vi "NXTMMX-DM.vi"(0 "Input of Motor Multiplexer":T4={"NXTMMX Address"=6, "Which Motor"=0, "Operation"=0, "Next Action"=0, "Position"=0, "Direction"=FALSE, "Power"=100, "Durartion"=0, "Wait for Completion"=FALSE, "Relative"=FALSE} {"Next Action" items=["Float", "Brake"]; "Operation" items=["Run Unlimited", "Run Seconds", "Run Tachometer"]; "Which Motor" items=["Motor 1", "Motor 2", "Both Motors"]; "NXTMMX Address" min=2 max=254 step=2 format="%x"}, 2 "NXT":T2={"Hardware"="NXT", "Flattened String"=""}, 3 "Input Port":T3 items=["Port 1", "Port 2", "Port 3", "Port 4"]) -> (1 "Output of Motor Multiplexer":T1, 4 "NXT dup":T2={"Hardware"="NXT", "Flattened String"=""})   [LabVIEW 2010]
uses:
  <vilib>/NXT/Block Support/NXT_InputPort.ctl
  <vilib>/NXT/Subs/LVHSConnector.ctl
  <vilib>/NXT/Block Support/HWPage.SensorType.ctl
  <vilib>/NXT/Block Support/HWPage.SensorMode.ctl
  <vilib>/NXT/Dual Mode Library/Waits/Wait_Num(msec).vi
panel:
  out "Address":i32
  # "mindsensors.com\nCopyright (c) 2009 by mindsensors.com\nEmail: info (<at>) mindsensors (<dot>) com\n\nThis program is free software. You can redistribute it and/or modify\nit under the terms of the GNU General Public License as published by\nthe Free Software Foundation; version 3 of the License.\nRead the license at: http://www.gnu.org/licenses/gpl.txt"
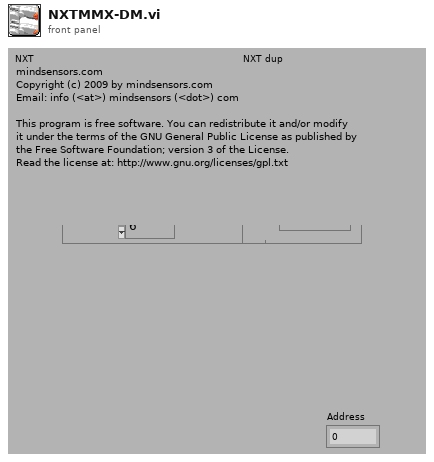
[diagram p1: front panel]
types:
  T1 = cluster{"Milivolts":u16, "Position 1":i32, "Position 2":i32, "Motor battery Voltage":dbl}
  T2 = typedef "LVHSConnector.ctl" = cluster{"Hardware":string, "Flattened String":string}
  T3 = typedef "NXT_InputPort.ctl" = u8
  T4 = cluster{"NXTMMX Address":u8, "Which Motor":u8, "Operation":u8, "Next Action":u8, "Position":i32, "Direction":bool, "Power":i8, "Durartion":u8, "Wait for Completion":bool, "Relative":bool}
  T5 = typedef "HWPage.SensorType.ctl" = u8
  T6 = typedef "HWPage.SensorMode.ctl" = u8
  T7 = cluster{"millivolts":i32, "(hi.lo)":u16, "(hi.lo)":u16, dbl}
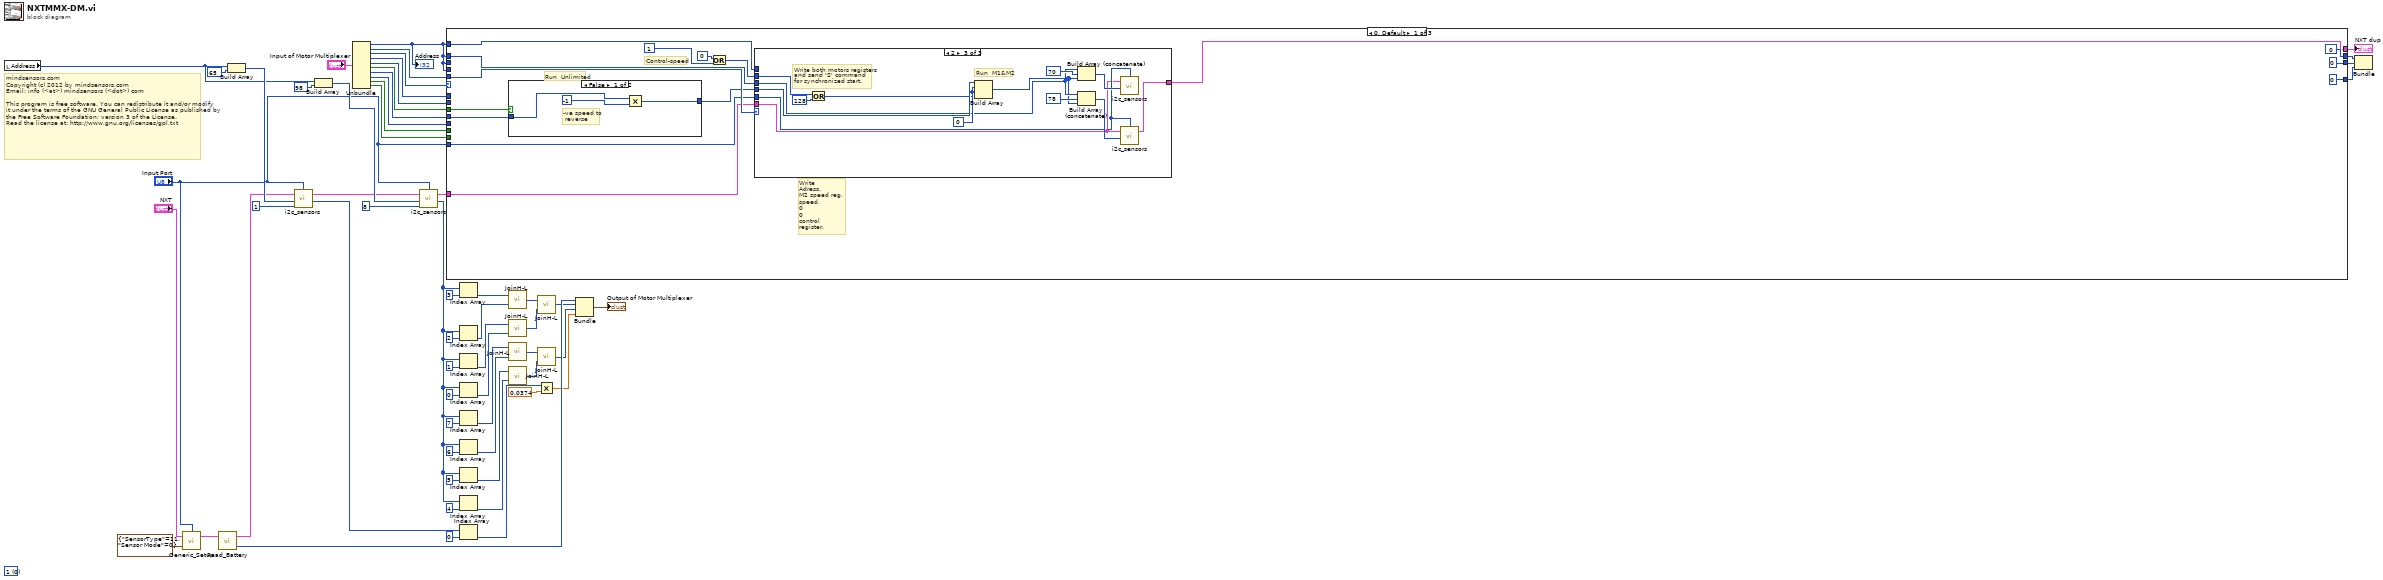
[diagram p0: block diagram]
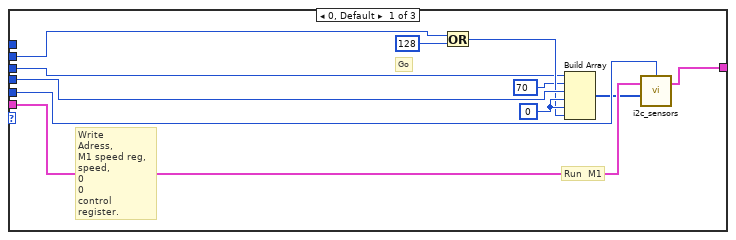
[diagram p2: hidden frame]
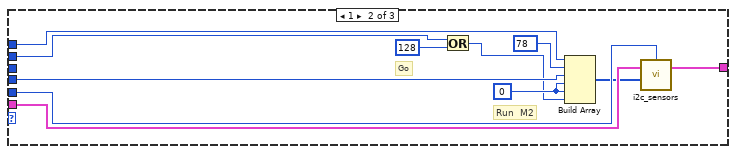
[diagram p3: hidden frame]
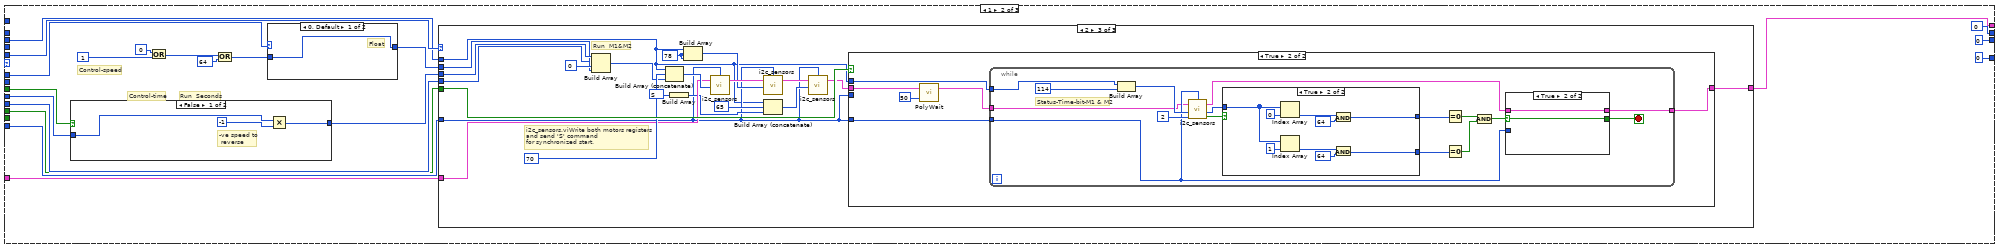
[diagram p5: hidden frame]
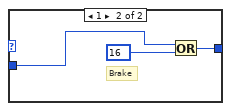
[diagram p6: hidden frame]
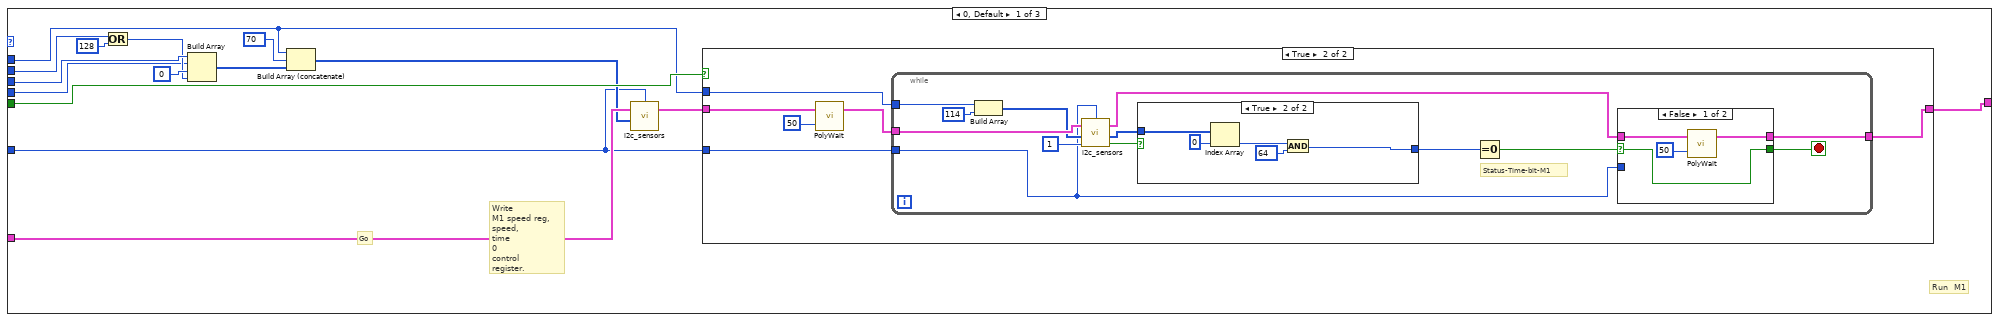
[diagram p7: hidden frame]
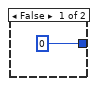
[diagram p10: hidden frame]
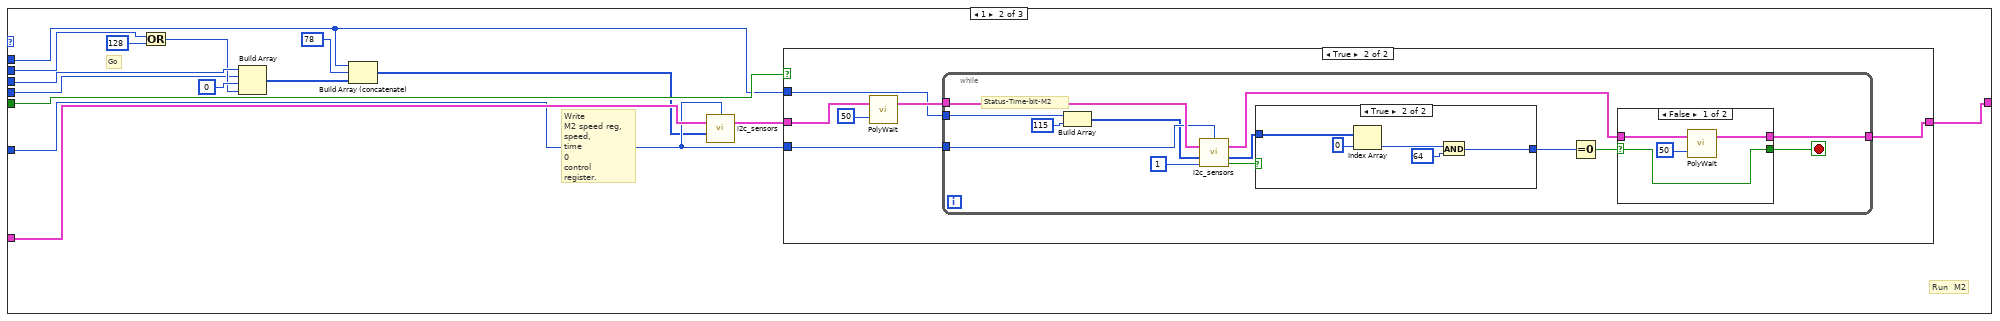
[diagram p11: hidden frame]
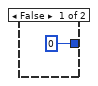
[diagram p14: hidden frame]
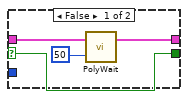
[diagram p16: hidden frame]
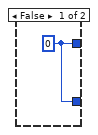
[diagram p17: hidden frame]
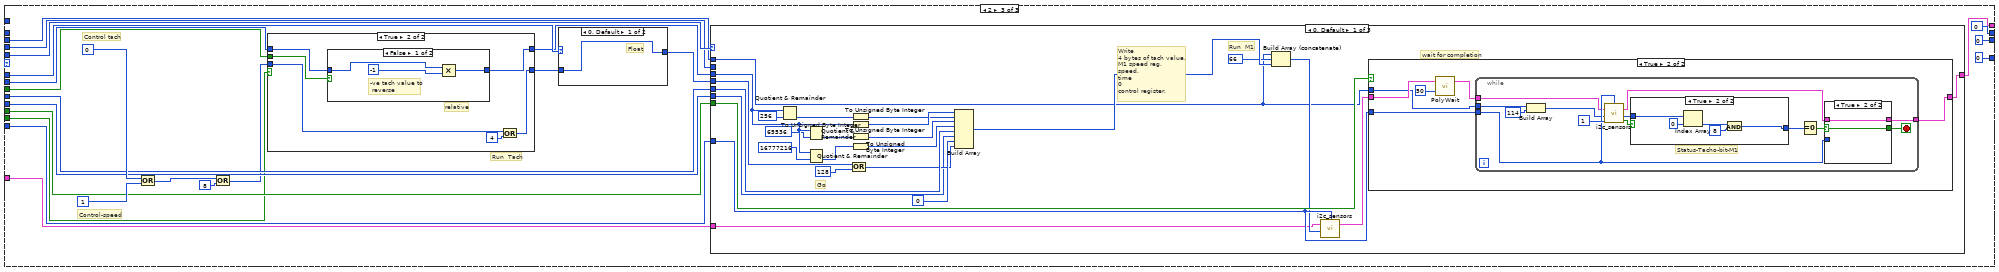
[diagram p19: hidden frame]
diagram:
  (unwired) i16 0 items=["1", "2", "3", "4", "5", "6", "7", "8"] ("Line")
  # "mindsensors.com\nCopyright (c) 2012 by mindsensors.com\nEmail: info (<at>) mindsensors (<dot>) com\n\nThis program is free software. You can redistribute it and/or modify\nit under the terms of the GNU General Public License as published by\nthe Free Software Foundation; version 3 of the License.\nRead the license at: http://www.gnu.org/licenses/gpl.txt"
  n1 = local read "Address"() -> (w4:i32)
  n2 = call <vilib>:"Generic_Setup.vi"("Sensor Setup"=cluster{"SensorType":T5, "Sensor Mode":T6} {"SensorType"=11, "Sensor Mode"=0}, "NXT"="NXT", "Port"="Input Port") -> ("NXT"=w49:T2)  [unwired: 1 out]
  n3 = call <vilib>:"Read_Battery.vi"("NXT"=w49) -> ("millivolts"=w23:i32, "NXT"=w3:T2)  [unwired: 2 in]
  n4 = Build Array(w4, u8 65 ("Reg Address")) -> (w35:i32[])
  n5 = call <vilib>:"i2c_sensors.vi"("Return Length"=u8 1 ("bytes to read"), "Bytes to Write"=w35, "NXT"=w3, "Port"="Input Port") -> ("Bytes read"=w34:u8[], "NXT"=w29:T2)  [unwired: 1 in, 1 out]
  n6 = Build Array(w4, u8 98 ("Reg Address")) -> (w33:i32[])
  n7 = Unbundle("Input of Motor Multiplexer") -> ("NXTMMX Address"=w51:u8, "Which Motor"=w53:u8, "Operation"=w58:u8, "Next Action"=w57:u8, "Position"=w55:i32, "Direction"=w54:bool, "Power"=w56:i8, "Durartion"=w52:u8, "Wait for Completion"=w25:bool, "Relative"=w24:bool)
  "Address" <- w51
  n8 = call <vilib>:"i2c_sensors.vi"("Return Length"=u8 8 ("bytes to read"), "Bytes to Write"=w33, "NXT"=w29, "Port"="Input Port") -> ("Bytes read"=w30:u8[], "NXT"=w27:T2)  [unwired: 1 in, 1 out]
  n9 = case shown="0, Default" w58 {
    tunnel: w54 -> [w72 w132 w318]
    tunnel: w56 -> [w71 w131 w308]
    tunnel: w53 -> [w70 w130 w317]
    tunnel: "Input Port" -> [w68 w128 w316]
    tunnel: w52 -> [_ w125 w313]
    tunnel: w57 -> [_ w124 w312]
    tunnel: w55 -> [_ _ w309]
    tunnel: w25 -> [_ w121 w310]
    tunnel: w24 -> [_ _ w306]
    tunnel: [0 0 0] -> w22
    tunnel: [u32 0 ("Out") u32 0 ("Out") u32 0 ("Out")] -> w21
    tunnel: [u16 0 u16 0 u16 0] -> w20
    tunnel: w27 -> [w63 w117 w299]
    tunnel: [w62 w116 w300] -> w19
    tunnel: w51 -> [_ w115 w298]
    tunnel: w51 -> [w61 _ _]
    tunnel: w51 -> [_ _ w297]
    tunnel: w51 -> [w60 _ _]
    frame 0, Default {
      # "Write\nAdress, \nM2 speed reg,\nspeed,\n0\n0\ncontrol register."
      # "Control-speed"
      # "Run  Unlimited"
      n10 = case shown="False" w72 {
        tunnel: w71 -> [w113 w114]
        tunnel: [w111 w114] -> w69
        frame False {
          # "-ve speed to\n reverse"
          n11 = Multiply(x=w113, y=i8 -1) -> (x*y=w111:i8)
        }
        frame True {
        }
      }
      n12 = Or(x=0, y=1) -> (x .or. y?=w67:i32)
      n13 = case shown="2" w70 {
        tunnel: w67 -> [w84 w95 w98]
        tunnel: w69 -> [w83 w94 w105]
        tunnel: w68 -> [w78 w91 w102]
        tunnel: w63 -> [w80 w90 w101]
        tunnel: [w79 w89 w100] -> w62
        tunnel: w61 -> [w77 _ w104]
        tunnel: w60 -> [_ w88 _]
        frame 0, Default {
          w82 = 0
          # "Go"
          # "Run  M1"
          # "Write \nAdress,\nM1 speed reg,\nspeed,\n0\n0\ncontrol register."
          n14 = Or(x=w84, y=128) -> (x .or. y?=w81:i32)
          n15 = Build Array(w77, 70, w83, w82, w82, w81) -> (w75:i32[])
          n16 = call <vilib>:"i2c_sensors.vi"("Bytes to Write"=w75, "NXT"=w80, "Port"=w78) -> ("NXT"=w79:T2)  [unwired: 2 in, 2 out]
        }
        frame 1 {
          w93 = 0
          # "Go"
          # "Run  M2"
          n17 = Or(x=w95, y=128) -> (x .or. y?=w92:i32)
          n18 = Build Array(w88, 78, w94, w93, w93, w92) -> (w86:i32[])
          n19 = call <vilib>:"i2c_sensors.vi"("Bytes to Write"=w86, "NXT"=w90, "Port"=w91) -> ("NXT"=w89:T2)  [unwired: 2 in, 2 out]
        }
        frame 2 {
          w106 = 0
          # "Write both motors registers\nand send 'S' command \nfor synchronized start."
          # "Run  M1&M2"
          n20 = Or(x=w98, y=128) -> (x .or. y?=w97:i32)
          n21 = Build Array(w105, w106, w106, w97) -> (w103:i32[])
          n22 = Build Array (concatenate)(w104, 70, w103) -> (w107:i32[])
          n23 = Build Array (concatenate)(w104, 78, w103) -> (w109:i32[])
          n24 = call <vilib>:"i2c_sensors.vi"("Bytes to Write"=w107, "NXT"=w101, "Port"=w102) -> ()  [unwired: 2 in, 3 out]
          n25 = call <vilib>:"i2c_sensors.vi"("Bytes to Write"=w109, "NXT"=w101, "Port"=w102) -> ("NXT"=w100:T2)  [unwired: 2 in, 2 out]
        }
      }
    }
    frame 1 {
      # "Control-time"
      # "Control-speed"
      # "Run  Seconds"
      n26 = case shown="False" w132 {
        tunnel: w131 -> [w295 w296]
        tunnel: [w293 w296] -> w129
        frame False {
          # "-ve speed to\n reverse"
          n27 = Multiply(x=w295, y=i8 -1) -> (x*y=w293:i8)
        }
        frame True {
        }
      }
      n28 = Or(x=0, y=1) -> (x .or. y?=w126:i32)
      n29 = Or(x=w126, y=64) -> (x .or. y?=w123:i32)
      n30 = case shown="0, Default" w124 {
        tunnel: w123 -> [w135 w137]
        tunnel: [w135 w138] -> w122
        frame 0, Default {
          # "Float"
        }
        frame 1 {
          # "Brake"
          n31 = Or(x=w137, y=16) -> (x .or. y?=w138:i32)
        }
      }
      n32 = case shown="2" w130 {
        tunnel: w122 -> [w152 w199 w250]
        tunnel: w129 -> [w151 w198 w253]
        tunnel: w128 -> [w141 w190 w235]
        tunnel: w125 -> [w148 w195 w249]
        tunnel: w121 -> [w147 w194 w248]
        tunnel: w117 -> [w145 w193 w244]
        tunnel: [w140 w187 w234] -> w116
        tunnel: w115 -> [w139 w186 w233]
        frame 0, Default {
          # "Go"
          # "Run  M1"
          # "Write \nM1 speed reg,\nspeed,\ntime\n0\ncontrol register."
          n33 = Or(x=w152, y=128) -> (x .or. y?=w149:i32)
          n34 = Build Array(w151, w148, 0, w149) -> (w142:i32[])
          n35 = Build Array (concatenate)(w139, 70, w142) -> (w144:i32[])
          n36 = call <vilib>:"i2c_sensors.vi"("Bytes to Write"=w144, "NXT"=w145, "Port"=w141) -> ("NXT"=w146:T2)  [unwired: 2 in, 2 out]
          n37 = case shown="True" w147 {
            tunnel: w141 -> [_ w160]
            tunnel: w146 -> [w154 w158]
            tunnel: [w154 w156] -> w140
            tunnel: w139 -> [_ w155]
            frame False {
            }
            frame True {
              n38 = call-poly <vilib>:"PolyWait.vi"("Time (100 msec)"=u16 50 ("Delay ms"), "NXT"=w158) -> ("NXT"=w157:T2)  [unwired: 2 in]
              n39 = while {
                tunnel: w160 -> [w164]
                tunnel: w157 -> [w169]
                tunnel: [w168] -> w156
                tunnel: w155 -> [w162]
                stop <- w172 stop-if-true
                # "Status-Time-bit-M1"
                n40 = Build Array(w162, 114) -> (w165:i32[])
                n41 = call <vilib>:"i2c_sensors.vi"("Return Length"=1, "Bytes to Write"=w165, "NXT"=w169, "Port"=w164) -> ("Success?"=w161:bool, "Bytes read"=w167:u8[], "NXT"=w170:T2)  [unwired: 1 in]
                n42 = case shown="True" w161 {
                  tunnel: w167 -> [_ w185]
                  tunnel: [u8 0 w181] -> w173
                  frame False {
                  }
                  frame True {
                    n43 = Index Array(array=w185, index=0) -> (element=w182:u8)
                    n44 = And(x=w182, y=u8 64) -> (x .and. y?=w181:u8)
                  }
                }
                n45 = Equal To 0?(x=w173) -> (x = 0?=w171:bool)
                n46 = case shown="False" w171 {
                  selector: w171 -> [w177 w179]
                  tunnel: w164 -> [_ _]
                  tunnel: [w177 w179] -> w172
                  tunnel: w170 -> [w175 w178]
                  tunnel: [w174 w178] -> w168
                  frame False {
                    n47 = call-poly <vilib>:"PolyWait.vi"("Time (100 msec)"=u16 50 ("Delay ms"), "NXT"=w175) -> ("NXT"=w174:T2)  [unwired: 2 in]
                  }
                  frame True {
                  }
                }
              }
            }
          }
        }
        frame 1 {
          # "Go"
          # "Run  M2"
          # "Write \nM2 speed reg,\nspeed,\ntime\n0\ncontrol register."
          n48 = Or(x=w199, y=128) -> (x .or. y?=w196:i32)
          n49 = Build Array(w198, w195, 0, w196) -> (w191:i32[])
          n50 = Build Array (concatenate)(w186, 78, w191) -> (w189:i32[])
          n51 = call <vilib>:"i2c_sensors.vi"("Bytes to Write"=w189, "NXT"=w193, "Port"=w190) -> ("NXT"=w188:T2)  [unwired: 2 in, 2 out]
          n52 = case shown="True" w194 {
            tunnel: w190 -> [_ w207]
            tunnel: w188 -> [w201 w205]
            tunnel: [w201 w203] -> w187
            tunnel: w186 -> [_ w202]
            frame False {
            }
            frame True {
              n53 = call-poly <vilib>:"PolyWait.vi"("Time (100 msec)"=u16 50 ("Delay ms"), "NXT"=w205) -> ("NXT"=w204:T2)  [unwired: 2 in]
              n54 = while {
                tunnel: w207 -> [w214]
                tunnel: w204 -> [w215]
                tunnel: [w217] -> w203
                tunnel: w202 -> [w209]
                stop <- w219 stop-if-true
                # "Status-Time-bit-M2"
                n55 = Build Array(w209, 115) -> (w211:i32[])
                n56 = call <vilib>:"i2c_sensors.vi"("Return Length"=1, "Bytes to Write"=w211, "NXT"=w215, "Port"=w214) -> ("Success?"=w208:bool, "Bytes read"=w210:u8[], "NXT"=w216:T2)  [unwired: 1 in]
                n57 = case shown="True" w208 {
                  tunnel: w210 -> [_ w232]
                  tunnel: [u8 0 w228] -> w220
                  frame False {
                  }
                  frame True {
                    n58 = Index Array(array=w232, index=0) -> (element=w229:u8)
                    n59 = And(x=w229, y=u8 64) -> (x .and. y?=w228:u8)
                  }
                }
                n60 = Equal To 0?(x=w220) -> (x = 0?=w218:bool)
                n61 = case shown="False" w218 {
                  selector: w218 -> [w224 w226]
                  tunnel: [w224 w226] -> w219
                  tunnel: [w222 w225] -> w217
                  tunnel: w216 -> [w221 w225]
                  frame False {
                    n62 = call-poly <vilib>:"PolyWait.vi"("Time (100 msec)"=u16 50 ("Delay ms"), "NXT"=w221) -> ("NXT"=w222:T2)  [unwired: 2 in]
                  }
                  frame True {
                  }
                }
              }
            }
          }
        }
        frame 2 {
          w251 = u16 83 items=["S"=83]
          w243 = 78
          # "i2c_sensors.viWrite both motors registers\nand send 'S' command \nfor synchronized start."
          # "Run  M1&M2"
          n63 = Build Array(w253, w249, 0, w250) -> (w246:i32[])
          n64 = Build Array (concatenate)(w233, 70, w246) -> (w245:i32[])
          n65 = Build Array(w251) -> (w241:u16[])
          n66 = Build Array(w233, w243, w243) -> (w238:i32[])
          n67 = call <vilib>:"i2c_sensors.vi"("Bytes to Write"=w245, "NXT"=w244, "Port"=w235) -> ("NXT"=w239:T2)  [unwired: 2 in, 2 out]
          n68 = call <vilib>:"i2c_sensors.vi"("Bytes to Write"=w238, "NXT"=w239, "Port"=w235) -> ("NXT"=w240:T2)  [unwired: 2 in, 2 out]
          n69 = Build Array (concatenate)(w233, 65, w241) -> (w237:i32[])
          n70 = call <vilib>:"i2c_sensors.vi"("Bytes to Write"=w237, "NXT"=w240, "Port"=w235) -> ("NXT"=w236:T2)  [unwired: 2 in, 2 out]
          n71 = case shown="True" w248 {
            tunnel: w235 -> [_ _]
            tunnel: w236 -> [w254 w259]
            tunnel: w235 -> [_ w257]
            tunnel: [w254 w256] -> w234
            tunnel: w233 -> [_ w255]
            frame False {
            }
            frame True {
              n72 = call-poly <vilib>:"PolyWait.vi"("Time (100 msec)"=u16 50 ("Delay ms"), "NXT"=w259) -> ("NXT"=w258:T2)  [unwired: 2 in]
              n73 = while {
                tunnel: w258 -> [w264]
                tunnel: w257 -> [w267]
                tunnel: [w263] -> w256
                tunnel: w255 -> [w262]
                stop <- w271 stop-if-true
                # "Status-Time-bit-M1 & M2"
                n74 = Build Array(w262, 114) -> (w268:i32[])
                n75 = call <vilib>:"i2c_sensors.vi"("Return Length"=2, "Bytes to Write"=w268, "NXT"=w264, "Port"=w267) -> ("Success?"=w261:bool, "Bytes read"=w266:u8[], "NXT"=w265:T2)  [unwired: 1 in]
                n76 = case shown="True" w261 {
                  tunnel: w266 -> [_ w291]
                  tunnel: [w283 w284] -> w276
                  tunnel: [w283 w286] -> w275
                  frame False {
                    w283 = u8 0
                  }
                  frame True {
                    n77 = Index Array(array=w291, index=0) -> (element=w287:u8)
                    n78 = Index Array(array=w291, index=1) -> (element=w285:u8)
                    n79 = And(x=w287, y=u8 64) -> (x .and. y?=w286:u8)
                    n80 = And(x=w285, y=u8 64) -> (x .and. y?=w284:u8)
                  }
                }
                n81 = Equal To 0?(x=w275) -> (x = 0?=w274:bool)
                n82 = Equal To 0?(x=w276) -> (x = 0?=w273:bool)
                n83 = And(x=w274, y=w273) -> (x .and. y?=w272:bool)
                n84 = case shown="True" w272 {
                  selector: w272 -> [w280 w282]
                  tunnel: w267 -> [_ _]
                  tunnel: [w280 w282] -> w271
                  tunnel: w265 -> [w278 w281]
                  tunnel: [w277 w281] -> w263
                  frame False {
                    n85 = call-poly <vilib>:"PolyWait.vi"("Time (100 msec)"=u16 50 ("Delay ms"), "NXT"=w278) -> ("NXT"=w277:T2)  [unwired: 2 in]
                  }
                  frame True {
                  }
                }
              }
            }
          }
        }
      }
    }
    frame 2 {
      # "Run  Tach"
      # "Control tach"
      # "Control-speed"
      n86 = Or(x=0, y=1) -> (x .or. y?=w314:i32)
      n87 = Or(x=w314, y=8) -> (x .or. y?=w305:i32)
      n88 = case shown="True" w306 {
        tunnel: w318 -> [_ w328]
        tunnel: w309 -> [w322 w327]
        tunnel: [w322 w326] -> w307
        tunnel: w305 -> [w321 w325]
        tunnel: [w321 w323] -> w304
        frame False {
          # "absolute\nignore the direction"
        }
        frame True {
          # "relative"
          n89 = case shown="False" w328 {
            tunnel: w327 -> [w331 w332]
            tunnel: [w329 w332] -> w326
            frame False {
              # "-ve tach value to\n reverse"
              n90 = Multiply(x=w331, y=i8 -1) -> (x*y=w329:i32)
            }
            frame True {
            }
          }
          n91 = Or(x=w325, y=4) -> (x .or. y?=w323:i32)
        }
      }
      n92 = case shown="0, Default" w312 {
        tunnel: [w333 w336] -> w311
        tunnel: w304 -> [w333 w334]
        frame 0, Default {
          # "Float"
        }
        frame 1 {
          # "Brake"
          n93 = Or(x=w334, y=16) -> (x .or. y?=w336:i32)
        }
      }
      n94 = case shown="0, Default" w317 {
        tunnel: w311 -> [w361 w419 w482]
        tunnel: w316 -> [w343 w400 w454]
        tunnel: w313 -> [w357 w415 w481]
        tunnel: w310 -> [w356 w414 w480]
        tunnel: w308 -> [w360 w418 w479]
        tunnel: w307 -> [w354 w407 w472]
        tunnel: [w337 w395 w467] -> w300
        tunnel: w299 -> [w340 w398 w466]
        tunnel: w298 -> [w338 _ _]
        tunnel: w297 -> [_ w396 _]
        frame 0, Default {
          # "wait for completion"
          # "Go"
          # "Run  M1"
          # "Write\n4 bytes of tach value. \nM1 speed reg,\nspeed,\ntime\n0\ncontrol register."
          n95 = Quotient & Remainder(x=w354, y=u32 256) -> (floor(x/y)=w350:u32)  [unwired: 1 out]
          n96 = Quotient & Remainder(x=w354, y=u32 65536) -> (floor(x/y)=w348:u32)  [unwired: 1 out]
          n97 = Quotient & Remainder(x=w354, y=u32 16777216) -> (floor(x/y)=w345:u32)  [unwired: 1 out]
          n98 = Or(x=w361, y=128) -> (x .or. y?=w358:i32)
          n99 = To Unsigned Byte Integer(number=w350) -> (unsigned 8bit integer=w349:u8)
          n100 = To Unsigned Byte Integer(number=w354) -> (unsigned 8bit integer=w355:u8)
          n101 = To Unsigned Byte Integer(number=w348) -> (unsigned 8bit integer=w347:u8)
          n102 = To Unsigned Byte Integer(number=w345) -> (unsigned 8bit integer=w346:u8)
          n103 = Build Array(w355, w349, w347, w346, w360, w357, 0, w358) -> (w344:i32[])
          n104 = Build Array (concatenate)(w338, 66, w344) -> (w341:i32[])
          n105 = call <vilib>:"i2c_sensors.vi"("Bytes to Write"=w341, "NXT"=w340, "Port"=w343) -> ("NXT"=w339:T2)  [unwired: 2 in, 2 out]
          n106 = case shown="True" w356 {
            tunnel: w343 -> [_ w369]
            tunnel: w339 -> [w363 w367]
            tunnel: w338 -> [_ w366]
            tunnel: [w363 w364] -> w337
            frame False {
            }
            frame True {
              n107 = call-poly <vilib>:"PolyWait.vi"("Time (100 msec)"=u16 50 ("Delay ms"), "NXT"=w367) -> ("NXT"=w365:T2)  [unwired: 2 in]
              n108 = while {
                tunnel: w369 -> [w377]
                tunnel: w366 -> [w375]
                tunnel: w365 -> [w374]
                tunnel: [w372] -> w364
                stop <- w380 stop-if-true
                # "Status-Tacho-bit-M1"
                n109 = Build Array(w375, 114) -> (w370:i32[])
                n110 = call <vilib>:"i2c_sensors.vi"("Return Length"=1, "Bytes to Write"=w370, "NXT"=w374, "Port"=w377) -> ("Success?"=w371:bool, "Bytes read"=w378:u8[], "NXT"=w373:T2)  [unwired: 1 in]
                n111 = case shown="True" w371 {
                  tunnel: w378 -> [_ w394]
                  tunnel: [u8 0 w390] -> w382
                  frame False {
                  }
                  frame True {
                    n112 = Index Array(array=w394, index=0) -> (element=w391:u8)
                    n113 = And(x=w391, y=u8 8) -> (x .and. y?=w390:u8)
                  }
                }
                n114 = Equal To 0?(x=w382) -> (x = 0?=w381:bool)
                n115 = case shown="True" w381 {
                  selector: w381 -> [w386 w388]
                  tunnel: w377 -> [_ _]
                  tunnel: [w386 w388] -> w380
                  tunnel: w373 -> [w384 w387]
                  tunnel: [w383 w387] -> w372
                  frame False {
                    n116 = call-poly <vilib>:"PolyWait.vi"("Time (100 msec)"=u16 50 ("Delay ms"), "NXT"=w384) -> ("NXT"=w383:T2)  [unwired: 2 in]
                  }
                  frame True {
                  }
                }
              }
            }
          }
        }
        frame 1 {
          # "Go"
          # "Run  M2"
          # "Write \nM2 speed reg,\nspeed,\ntime\n0\ncontrol register."
          n117 = Quotient & Remainder(x=w407, y=u32 256) -> (floor(x/y)=w410:u32)  [unwired: 1 out]
          n118 = Quotient & Remainder(x=w407, y=u32 65536) -> (floor(x/y)=w409:u32)  [unwired: 1 out]
          n119 = Quotient & Remainder(x=w407, y=u32 16777216) -> (floor(x/y)=w408:u32)  [unwired: 1 out]
          n120 = Or(x=w419, y=128) -> (x .or. y?=w416:i32)
          n121 = To Unsigned Byte Integer(number=w410) -> (unsigned 8bit integer=w405:u8)
          n122 = To Unsigned Byte Integer(number=w407) -> (unsigned 8bit integer=w406:u8)
          n123 = To Unsigned Byte Integer(number=w409) -> (unsigned 8bit integer=w404:u8)
          n124 = To Unsigned Byte Integer(number=w408) -> (unsigned 8bit integer=w403:u8)
          n125 = Build Array(w406, w405, w404, w403, w418, w415, 0, w416) -> (w401:i32[])
          n126 = Build Array (concatenate)(w396, 74, w401) -> (w399:i32[])
          n127 = call <vilib>:"i2c_sensors.vi"("Bytes to Write"=w399, "NXT"=w398, "Port"=w400) -> ("NXT"=w397:T2)  [unwired: 2 in, 2 out]
          n128 = case shown="True" w414 {
            tunnel: w400 -> [_ w427]
            tunnel: w397 -> [w421 w425]
            tunnel: w396 -> [_ w423]
            tunnel: [w421 w422] -> w395
            frame False {
            }
            frame True {
              n129 = call-poly <vilib>:"PolyWait.vi"("Time (100 msec)"=u16 50 ("Delay ms"), "NXT"=w425) -> ("NXT"=w424:T2)  [unwired: 2 in]
              n130 = while {
                tunnel: w427 -> [w431]
                tunnel: w424 -> [w437]
                tunnel: w423 -> [w435]
                tunnel: [w428] -> w422
                stop <- w438 stop-if-true
                # "Status-Tacho-bit-M2"
                n131 = Build Array(w435, 115) -> (w433:i32[])
                n132 = call <vilib>:"i2c_sensors.vi"("Return Length"=1, "Bytes to Write"=w433, "NXT"=w437, "Port"=w431) -> ("Success?"=w430:bool, "Bytes read"=w432:u8[], "NXT"=w429:T2)  [unwired: 1 in]
                n133 = case shown="True" w430 {
                  tunnel: w432 -> [_ w452]
                  tunnel: [u8 0 w448] -> w440
                  frame False {
                  }
                  frame True {
                    n134 = Index Array(array=w452, index=0) -> (element=w450:u8)
                    n135 = And(x=w450, y=u8 8) -> (x .and. y?=w448:u8)
                  }
                }
                n136 = Equal To 0?(x=w440) -> (x = 0?=w439:bool)
                n137 = case shown="True" w439 {
                  selector: w439 -> [w444 w446]
                  tunnel: w431 -> [_ _]
                  tunnel: [w444 w446] -> w438
                  tunnel: w429 -> [w442 w445]
                  tunnel: [w441 w445] -> w428
                  frame False {
                    n138 = call-poly <vilib>:"PolyWait.vi"("Time (100 msec)"=u16 50 ("Delay ms"), "NXT"=w442) -> ("NXT"=w441:T2)  [unwired: 2 in]
                  }
                  frame True {
                  }
                }
              }
            }
          }
        }
        frame 2 {
          w483 = u16 83 items=["S"=83]
          # "Write both motors registers\nand send 'S' command \nfor synchronized start."
          # "Run  M1&M2"
          n139 = Quotient & Remainder(x=w472, y=u32 256) -> (floor(x/y)=w475:u32)  [unwired: 1 out]
          n140 = Quotient & Remainder(x=w472, y=u32 65536) -> (floor(x/y)=w474:u32)  [unwired: 1 out]
          n141 = Quotient & Remainder(x=w472, y=u32 16777216) -> (floor(x/y)=w473:u32)  [unwired: 1 out]
          n142 = To Unsigned Byte Integer(number=w475) -> (unsigned 8bit integer=w470:u8)
          n143 = To Unsigned Byte Integer(number=w472) -> (unsigned 8bit integer=w471:u8)
          n144 = To Unsigned Byte Integer(number=w474) -> (unsigned 8bit integer=w469:u8)
          n145 = To Unsigned Byte Integer(number=w473) -> (unsigned 8bit integer=w468:u8)
          n146 = local read "Address"() -> (w453:i32)
          n147 = Build Array(w471, w470, w469, w468, w479, w481, 0, w482) -> (w457:i32[])
          n148 = Build Array (concatenate)(w453, 74, w457) -> (w462:i32[])
          n149 = Build Array (concatenate)(w453, 66, w457) -> (w460:i32[])
          n150 = Build Array(w483) -> (w455:u16[])
          n151 = call <vilib>:"i2c_sensors.vi"("Bytes to Write"=w460, "NXT"=w466, "Port"=w454) -> ("NXT"=w463:T2)  [unwired: 2 in, 2 out]
          n152 = call <vilib>:"i2c_sensors.vi"("Bytes to Write"=w462, "NXT"=w463, "Port"=w454) -> ("NXT"=w464:T2)  [unwired: 2 in, 2 out]
          n153 = Build Array (concatenate)(w453, 65, w455) -> (w461:i32[])
          n154 = call <vilib>:"i2c_sensors.vi"("Bytes to Write"=w461, "NXT"=w464, "Port"=w454) -> ("NXT"=w465:T2)  [unwired: 2 in, 2 out]
          n155 = case shown="True" w480 {
            tunnel: w454 -> [_ w491]
            tunnel: w465 -> [w485 w489]
            tunnel: [w485 w488] -> w467
            tunnel: w453 -> [_ w486]
            frame False {
            }
            frame True {
              n156 = call-poly <vilib>:"PolyWait.vi"("Time (100 msec)"=u16 50 ("Delay ms"), "NXT"=w489) -> ("NXT"=w487:T2)  [unwired: 2 in]
              n157 = while {
                tunnel: w491 -> [w496]
                tunnel: [w501] -> w488
                tunnel: w487 -> [w495]
                tunnel: w486 -> [w493]
                stop <- w502 stop-if-true
                # "Status-Tacho-bit-M1 & M2"
                n158 = Build Array(w493, 114) -> (w500:i32[])
                n159 = call <vilib>:"i2c_sensors.vi"("Return Length"=2, "Bytes to Write"=w500, "NXT"=w495, "Port"=w496) -> ("Success?"=w492:bool, "Bytes read"=w497:u8[], "NXT"=w494:T2)  [unwired: 1 in]
                n160 = case shown="True" w492 {
                  tunnel: w497 -> [_ w522]
                  tunnel: [w514 w515] -> w507
                  tunnel: [w514 w517] -> w506
                  frame False {
                    w514 = u8 0
                  }
                  frame True {
                    n161 = Index Array(array=w522, index=0) -> (element=w518:u8)
                    n162 = Index Array(array=w522, index=1) -> (element=w516:u8)
                    n163 = And(x=w518, y=u8 8) -> (x .and. y?=w517:u8)
                    n164 = And(x=w516, y=u8 8) -> (x .and. y?=w515:u8)
                  }
                }
                n165 = Equal To 0?(x=w506) -> (x = 0?=w505:bool)
                n166 = Equal To 0?(x=w507) -> (x = 0?=w504:bool)
                n167 = And(x=w505, y=w504) -> (x .and. y?=w503:bool)
                n168 = case shown="True" w503 {
                  selector: w503 -> [w511 w513]
                  tunnel: w496 -> [_ _]
                  tunnel: [w511 w513] -> w502
                  tunnel: [w509 w512] -> w501
                  tunnel: w494 -> [w508 w512]
                  frame False {
                    n169 = call-poly <vilib>:"PolyWait.vi"("Time (100 msec)"=u16 50 ("Delay ms"), "NXT"=w508) -> ("NXT"=w509:T2)  [unwired: 2 in]
                  }
                  frame True {
                  }
                }
              }
            }
          }
        }
      }
    }
  }
  "NXT dup" <- w19
  n170 = Index Array(array=w30, index=3) -> (element=w18:u8)
  n171 = Index Array(array=w30, index=2) -> (element=w17:u8)
  n172 = Index Array(array=w30, index=1) -> (element=w16:u8)
  n173 = Index Array(array=w30, index=0) -> (element=w15:u8)
  n174 = Index Array(array=w30, index=7) -> (element=w14:u8)
  n175 = Index Array(array=w30, index=6) -> (element=w13:u8)
  n176 = Index Array(array=w30, index=5) -> (element=w12:u8)
  n177 = Index Array(array=w30, index=4) -> (element=w11:u8)
  n178 = Index Array(array=w34, index=0) -> (element=w39:u8)
  n179 = call <vilib>:"JoinH-L.vi"("low"=w17, "hi"=w18) -> ("(hi.lo)"=w7:u16)
  n180 = call <vilib>:"JoinH-L.vi"("low"=w15, "hi"=w16) -> ("(hi.lo)"=w6:u16)
  n181 = call <vilib>:"JoinH-L.vi"("low"=w13, "hi"=w14) -> ("(hi.lo)"=w10:u16)
  n182 = call <vilib>:"JoinH-L.vi"("low"=w11, "hi"=w12) -> ("(hi.lo)"=w9:u16)
  n183 = call <vilib>:"JoinH-L.vi"("low"=w6, "hi"=w7) -> ("(hi.lo)"=w1:u16)
  n184 = call <vilib>:"JoinH-L.vi"("low"=w9, "hi"=w10) -> ("(hi.lo)"=w8:u16)
  n185 = Multiply(x=w39, y=0.0374) -> (x*y=w2:dbl)
  n186 = Bundle("millivolts"=w23, "(hi.lo)"=w1, "(hi.lo)"=w8, w2) -> (→"Output of Motor Multiplexer":T7)  [unwired: 1 in]
  n187 = Bundle(w22, "Out"=w21, w20) -> ()  [unwired: 1 in, 1 out]
